vi "Lambda Genesys Device Properties.vi"() -> ()   [LabVIEW 2011, in "Lambda Genesys2 Custom Device.lvlib"]
uses:
  Lambda Genesys2 Custom Device.lvlib
panel:
  in  "Baud Rate":string="Baud Rate"
  in  "Address":string="Address"
  in  "Resource":string="VISA Resource"
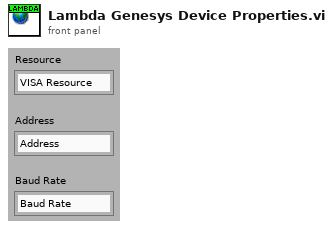
[diagram p1: front panel]
diagram:
